vi "GoV2.vi"(8 "Initial Coordinates":dbl[](array[numeric]), 9 "Timing Data":dbl[](array[numeric]), 10 "Control In":T1, 11 "Sensor Dispense in":refnum<class "Sensor Dispense.lvclass">) -> (2 "Control Out":T1, 3 "Sensor Dispense out":refnum<class "Sensor Dispense.lvclass">)   [LabVIEW 2020]
uses:
  Classes/Controller/I-O/I-O.lvclass
  Classes/Controller/Dispenser/Dispenser.lvclass
  C:/Program Files (x86)/Aerotech/A3200/LabVIEW/2010/Bin/Aerotech.A3200.dll
  Program Files (x86)/Aerotech/A3200/LabVIEW/2010/Bin/Aerotech.A3200.dll
  Classes/Controller/Controllers.ctl
  Classes/Controller/Controller.lvclass
  Sensor Dispense.lvclass
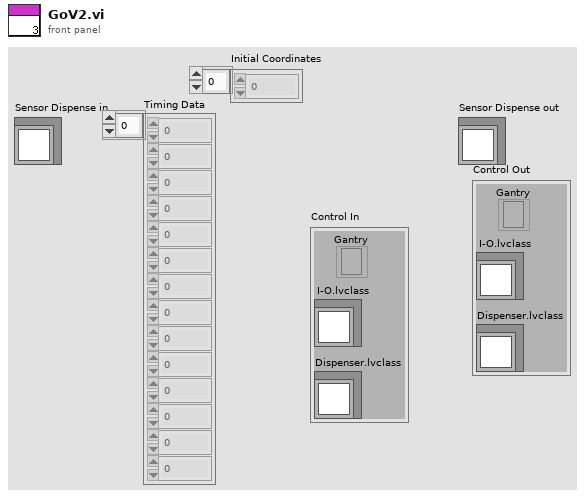
[diagram p1: front panel]
types:
  T1 = typedef "Controller.lvclass/Controllers.ctl" = cluster{"I-O.lvclass":refnum<class "I-O.lvclass">, "Dispenser.lvclass":refnum<class "Dispenser.lvclass">, "Gantry":refnum<k24>}
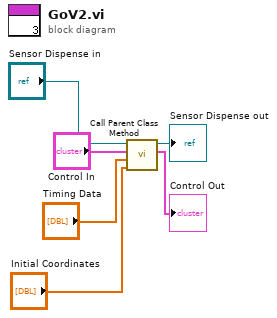
[diagram p0: block diagram]
diagram:
  n1 = call-parent "Call Parent Class Method"("Initial Coordinates"="Initial Coordinates", "Timing Data"="Timing Data", "Control In"="Control In", "Dispense in"="Sensor Dispense in") -> ("Control Out"=→"Control Out":T1, "Dispense out"=→"Sensor Dispense out":refnum<class "Sensor Dispense.lvclass">)  [unwired: 6 in]
